vi "OPTICAL_IN_TESTS.vi"(2 "connection ID CC":refnum<k5>, 3 "Chopper Serial Number":string="26") -> (0 "PASS / FAIL":bool, 1 "concatenated string":string)   [LabVIEW 2013]
panel:
  out "PROGRESS":i32(slide) scale=0.0..4.0
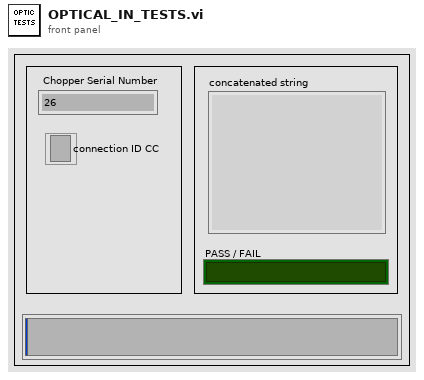
[diagram p1: front panel]
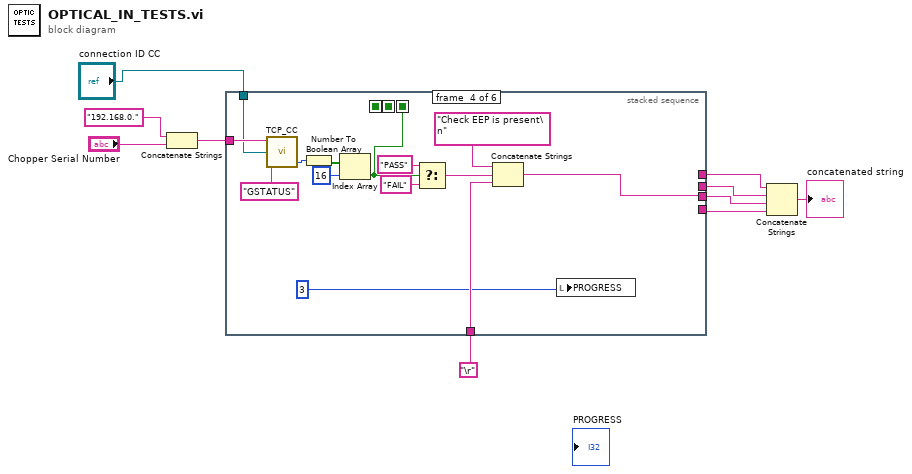
[diagram p0: block diagram]
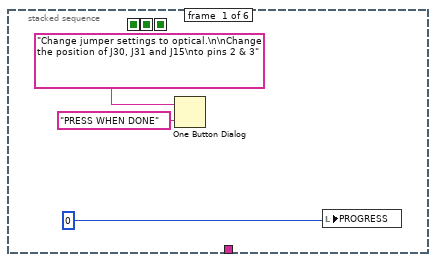
[diagram p2: hidden frame]
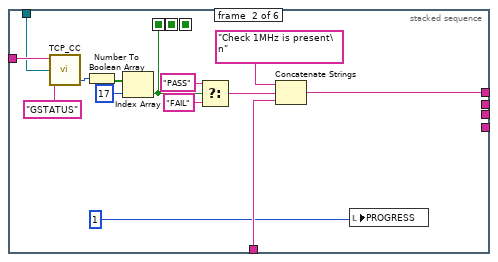
[diagram p3: hidden frame]
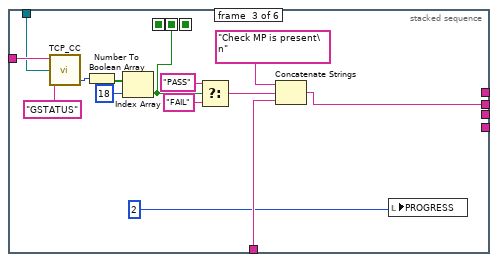
[diagram p4: hidden frame]
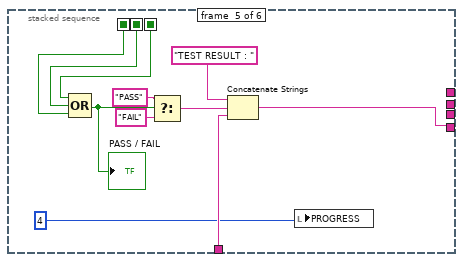
[diagram p5: hidden frame]
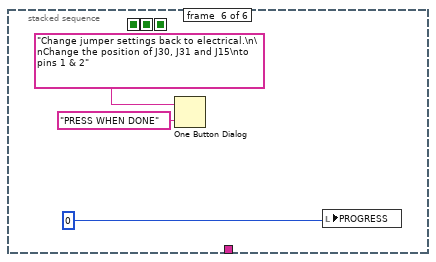
[diagram p6: hidden frame]
diagram:
  n1 = Concatenate Strings("192.168.0.", "Chopper Serial Number") -> (w8:string)
  n2 = stacked-sequence {
    seq-local: [_ w16 _ _ _ _] -> [_ _ _ _ w60 _]
    seq-local: [_ _ w30 _ _ _] -> [_ _ _ _ w61 _]
    seq-local: [_ _ _ w44 _ _] -> [_ _ _ _ w62 _]
    tunnel: w8 -> [_ w23 w37 w51 _ _]
    tunnel: "\r" -> [_ w18 w32 w46 w57 _]
    tunnel: [_ w17 _ _ _ _] -> w6
    tunnel: [_ _ w31 _ _ _] -> w5
    tunnel: [_ _ _ w45 _ _] -> w4
    tunnel: [_ _ _ _ w58 _] -> w3
    tunnel: "connection ID CC" -> [_ w14 w28 w42 _ _]
    frame #0 {
      n3 = One Button Dialog(message="Change jumper settings to optical.\n\nChange the position of J30, J31 and J15\nto pins 2 & 3", button name ("OK")="PRESS WHEN DONE") -> ()  [unwired: 1 out]
      n4 = local write "PROGRESS"(0) -> ()
    }
    frame #1 {
      n5 = call "TCP_CC.vi"("COMMAND"="GSTATUS", "connection ID"=w14, "IP ADDRESS"=w23) -> ("number"=w26:u32)  [unwired: 2 out]
      n6 = Number To Boolean Array(number=w26) -> (Boolean array=w25:bool[])
      n7 = Index Array(array=w25, index=17) -> (element=w16:bool)
      n8 = Select(t="PASS", s=w16, f="FAIL") -> (s? t:f=w19:string)
      n9 = Concatenate Strings("Check 1MHz is present\n", w19, w18) -> (w17:string)
      n10 = local write "PROGRESS"(1) -> ()
    }
    frame #2 {
      n11 = call "TCP_CC.vi"("COMMAND"="GSTATUS", "connection ID"=w28, "IP ADDRESS"=w37) -> ("number"=w40:u32)  [unwired: 2 out]
      n12 = Number To Boolean Array(number=w40) -> (Boolean array=w39:bool[])
      n13 = Index Array(array=w39, index=18) -> (element=w30:bool)
      n14 = Select(t="PASS", s=w30, f="FAIL") -> (s? t:f=w33:string)
      n15 = Concatenate Strings("Check MP is present\n", w33, w32) -> (w31:string)
      n16 = local write "PROGRESS"(2) -> ()
    }
    frame #3 {
      n17 = call "TCP_CC.vi"("COMMAND"="GSTATUS", "connection ID"=w42, "IP ADDRESS"=w51) -> ("number"=w54:u32)  [unwired: 2 out]
      n18 = Number To Boolean Array(number=w54) -> (Boolean array=w53:bool[])
      n19 = Index Array(array=w53, index=16) -> (element=w44:bool)
      n20 = Select(t="PASS", s=w44, f="FAIL") -> (s? t:f=w47:string)
      n21 = Concatenate Strings("Check EEP is present\n", w47, w46) -> (w45:string)
      n22 = local write "PROGRESS"(3) -> ()
    }
    frame #4 {
      n23 = Compound Arithmetic op=OR(w62, w61, w60) -> (w59:bool)
      "PASS / FAIL" <- w59
      n24 = Select(t="PASS", s=w59, f="FAIL") -> (s? t:f=w64:string)
      n25 = Concatenate Strings("TEST RESULT : ", w64, w57) -> (w58:string)
      n26 = local write "PROGRESS"(4) -> ()
    }
    frame #5 {
      n27 = One Button Dialog(message="Change jumper settings back to electrical.\n\nChange the position of J30, J31 and J15\nto pins 1 & 2", button name ("OK")="PRESS WHEN DONE") -> ()  [unwired: 1 out]
      n28 = local write "PROGRESS"(0) -> ()
    }
  }
  n29 = Concatenate Strings(w6, w5, w4, w3) -> (→"concatenated string":string)
